vi "Send FlushAppenderMsg.vi"(8 "error in (no error)":errorcluster, 10 "replyEnqueuer":refnum<class "Message Enqueuer.lvclass">, 11 "Enqueuer in":refnum<class "Message Enqueuer.lvclass">) -> (0 "error out":errorcluster, 3 "Enqueuer out":refnum<class "Message Enqueuer.lvclass">)   [LabVIEW 2026, in "Lumberjack.lvlib" / "FlushAppenderMsg.lvclass"]
doc: "Constructs a FlushAppenderMsg (payload-free) and enqueues it to an appender actor to force it to flush its sink.\nSent by the manager's BeginFlushDrain to every registered appender; the appender drains its statement queue, flushes (FlushSink), then replies with a FlushAckMsg (SRS-LMBR-002).\nLumberjack.lvlib, FlushAppenderMsg.lvclass, public."
uses:
  FlushAppenderMsg.lvclass
  <vilib>/ActorFramework/Message Enqueuer/Message Enqueuer.lvclass
  FlushAppenderMsg.lvclass/FlushAppenderMsg.ctl
  <vilib>/ActorFramework/Message Enqueuer/Message Enqueuer.lvclass/Message Enqueuer.ctl
  <vilib>/ActorFramework/Message Priority Queue/Priority Enqueue.vi
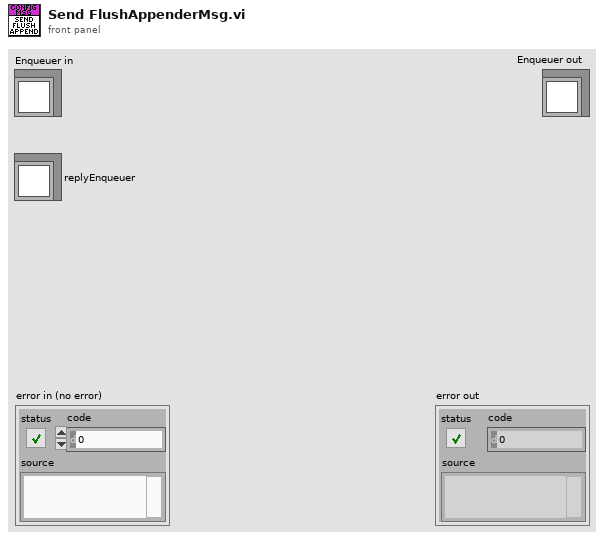
[diagram p1: front panel]
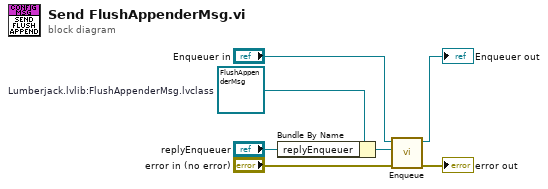
[diagram p0: block diagram]
diagram:
  w3 = refnum<class "FlushAppenderMsg.lvclass"> refnum  # Lumberjack.lvlib:FlushAppenderMsg.lvclass
  n1 = Bundle By Name(cluster=w3, "replyEnqueuer"="replyEnqueuer") -> (w2:refnum<class "FlushAppenderMsg.lvclass">)
  n2 = call <vilib>:"Enqueue.vi"("error in (no error)"="error in (no error)", "Message"=w2, "Message Enqueuer in"="Enqueuer in") -> ("error out"=→"error out":errorcluster, "Message Enqueuer out"=→"Enqueuer out":refnum<class "Message Enqueuer.lvclass">)  [unwired: 7 in]
